vi "Initialize.vi"(8 "error in (no error)":errorcluster, 9 "Reset (True)":bool=TRUE, 10 "ID Query (True)":bool=TRUE, 11 "VISA resource name":refnum<visa-resource-name>) -> (0 "error out":errorcluster, 3 "VISA resource name out":refnum<visa-resource-name>)   [LabVIEW 2018, in "Keithley DMM7512.lvlib"]
doc: "Establishes communication with the instrument and optionally performs an instrument identification query and/or an instrument reset. It also places the instrument in a default state needed for other instrument driver operations. Therefore, call this VI before calling other instrument driver VIs for this instrument. Generally, you need to call the Initialize VI only once at the beginning of an application."
uses:
  <instrlib>/Keithley DMM7512/Keithley DMM7512.lvlib
panel:
  # "(c) 2019 Keithley.  ALL RIGHTS RESERVED."
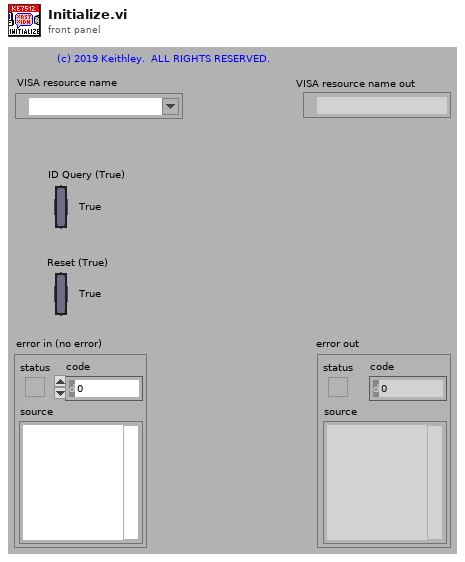
[diagram p1: front panel]
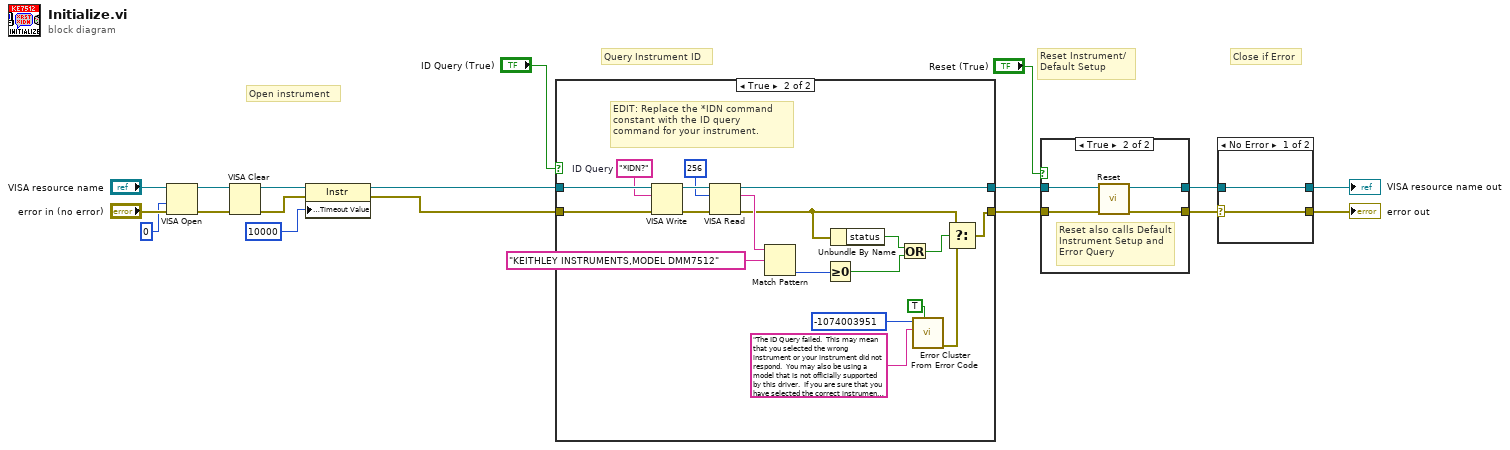
[diagram p0: block diagram]
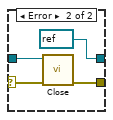
[diagram p2: hidden frame]
diagram:
  # "Close if Error"
  # "Query Instrument ID"
  # "Reset Instrument/\nDefault Setup"
  # "Open instrument"
  n1 = VISA Open(access mode=u32 0, error in (no error)="error in (no error)", VISA resource name="VISA resource name") -> (VISA resource name=w10:refnum<visa-resource-name>, error out=w9:errorcluster)  [unwired: 2 in]
  n2 = VISA Clear(VISA resource name=w10, error in (no error)=w9) -> (VISA resource name out=w8:refnum<visa-resource-name>, error out=w7:errorcluster)
  n3 = property class="Instr"(reference=w8, error in=w7, "General Settings:Timeout Value"=u32 10000) -> (reference out=w2:refnum<visa-resource-name>, error out=w1:errorcluster)
  n4 = case shown="True" "ID Query (True)" {
    tunnel: [w19 w39] -> w17
    tunnel: [w20 w36] -> w18
    tunnel: w2 -> [w20 w37]
    tunnel: w1 -> [w19 w38]
    frame False {
    }
    frame True {
      w30 = "*IDN?"  # ID Query
      # "EDIT: Replace the *IDN command\nconstant with the ID query\ncommand for your instrument."
      n5 = VISA Write(VISA resource name=w37, write buffer=w30, error in (no error)=w38) -> (VISA resource name out=w34:refnum<visa-resource-name>, error out=w33:errorcluster)  [unwired: 1 out]
      n6 = VISA Read(VISA resource name=w34, byte count=u32 256, error in (no error)=w33) -> (VISA resource name out=w36:refnum<visa-resource-name>, read buffer=w35:string, error out=w24:errorcluster)  [unwired: 1 out]
      n7 = Match Pattern(string=w35, regular expression="KEITHLEY INSTRUMENTS,MODEL DMM7512") -> (offset past match=w25:i32)  [unwired: 1 in, 3 out]
      n8 = Greater Or Equal To 0?(x=w25) -> (x >= 0?=w22:bool)
      n9 = Unbundle By Name(w24) -> ("status"=w23:bool)
      n10 = Or(x=w23, y=w22) -> (x .or. y?=w21:bool)
      n11 = call <vilib>:"Error Cluster From Error Code.vi"("show call chain? (False)"=TRUE, "error message (\"\")"="The ID Query failed.  This may mean that you selected the wrong instrument or your instrument did not respond.  You may also be using a model that is not officially supported by this driver.  If you are sure that you have selected the correct instrument and it is responding, try disabling the ID Query." ("Source (VI Name)"), "error code (0)"=-1074003951 ("Code")) -> ("error out"=w29:errorcluster)  [unwired: 6 in]
      n12 = Select(t=w24, s=w21, f=w29) -> (s? t:f=w39:errorcluster)
    }
  }
  n13 = case shown="True" "Reset (True)" {
    tunnel: w17 -> [w40 w42]
    tunnel: [w40 w45] -> w3
    tunnel: w18 -> [w41 w43]
    tunnel: [w41 w44] -> w4
    frame False {
    }
    frame True {
      # "Reset also calls Default Instrument Setup and Error Query"
      n14 = call <instrlib>:"Reset.vi"("error in (no error)"=w42, "VISA resource name"=w43) -> ("error out"=w45:errorcluster, "VISA resource name out"=w44:refnum<visa-resource-name>)  [unwired: 8 in]
    }
  }
  n15 = case shown="No Error" w3 {
    selector: w3 -> [w46 w49]
    tunnel: w4 -> [w47 w50]
    tunnel: [w47 refnum<visa-resource-name> refnum ("VISA resource name out")] -> w6
    tunnel: [w46 w51] -> w5
    frame No Error {
    }
    frame Error {
      n16 = call <instrlib>:"Close.vi"("error in (no error)"=w49, "VISA resource name"=w50) -> ("error out"=w51:errorcluster)  [unwired: 9 in]
    }
  }
  "VISA resource name out" <- w6
  "error out" <- w5
